vi "rmSharedMemory.vi"(8 "error in (no error)":errorcluster, 11 "SalProcess in":refnum<class "SalProcess.lvclass">) -> (0 "error out":errorcluster, 2 "outputMsg":string, 3 "SalProcess out":refnum<class "SalProcess.lvclass">)   [LabVIEW 2018, in "SalProcess.lvclass"]
doc: "Remove the shared memory of commandable SAL component (CSC)."
uses:
  SalProcess.lvclass
  SalProcess.lvclass/SalProcess.ctl
  LibReader/LibReader.lvclass/LibReader.ctl
  LibReader/LibReader.lvclass
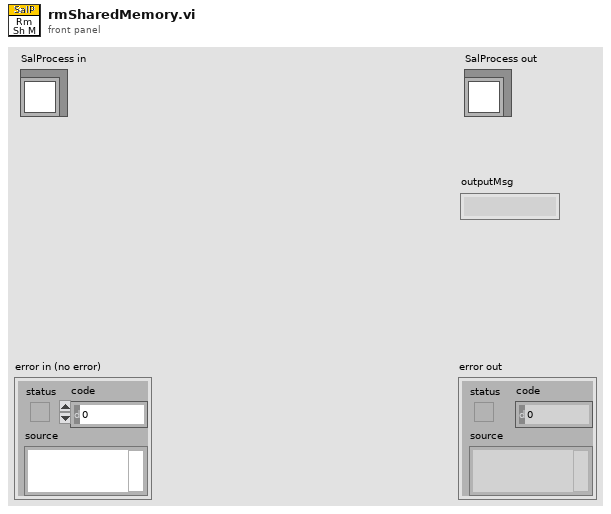
[diagram p1: front panel]
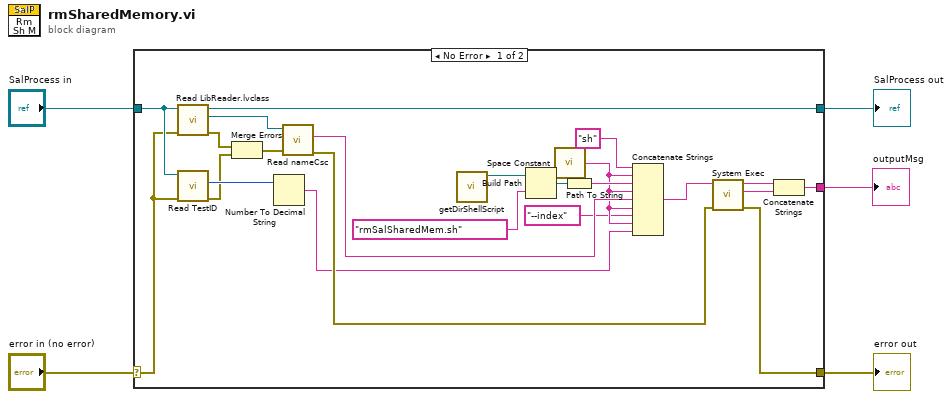
[diagram p0: block diagram]
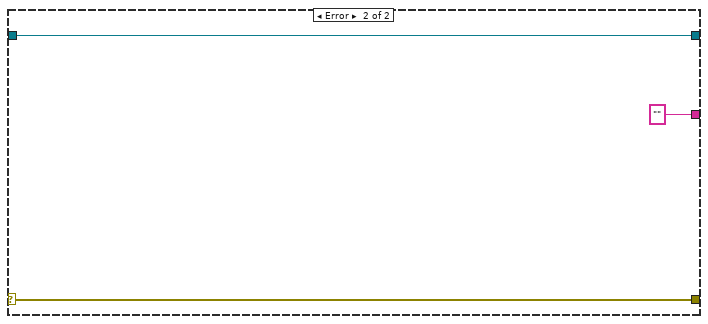
[diagram p2: hidden frame]
diagram:
  n1 = case shown="No Error" "error in (no error)" {
    selector: "error in (no error)" -> [w11 w31]
    tunnel: [w24 w31] -> w4
    tunnel: [w18 w30] -> w2
    tunnel: "SalProcess in" -> [w12 w30]
    tunnel: [w19 ""] -> w1
    frame No Error {
      n2 = call "Read LibReader.lvclass.vi"("error in (no error)"=w11, "SalProcess in"=w12) -> ("error out"=w7:errorcluster, "LibReader.lvclass"=w17:refnum<class "LibReader.lvclass">, "SalProcess out"=w18:refnum<class "SalProcess.lvclass">)  [unwired: 7 in]
      n3 = call "Read TestID.vi"("error in (no error)"=w11, "SalProcess in"=w12) -> ("error out"=w6:errorcluster, "TestID"=w10:i32)  [unwired: 7 in, 1 out]
      n4 = Merge Errors(w7, w6) -> (w8:errorcluster)
      n5 = Number To Decimal String(number=w10) -> (decimal integer string=w9:string)  [unwired: 1 in]
      n6 = call "Read nameCsc.vi"("error in (no error)"=w8, "LibReader in"=w17) -> ("error out"=w15:errorcluster, "nameCsc"=w16:string)  [unwired: 7 in, 1 out]
      n7 = call "getDirShellScript.vi"() -> ("dirShellScript"=w28:path)  [unwired: 11 in]
      n8 = Build Path(base path=w28, name or relative path="rmSalSharedMem.sh") -> (appended path=w26:path)
      n9 = call <vilib>:"Space Constant.vi"() -> ("String"=w14:string)
      n10 = Path To String(path=w26) -> (string=w25:string)
      n11 = Concatenate Strings("sh" ("string"), w14, w25, w14, w16, w14, "--index", w14, w9) -> (w22:string)
      n12 = call <vilib>:"System Exec.vi"("error in (no error)"=w15, "command line"=w22) -> ("error out"=w24:errorcluster, "standard error"=w20:string, "standard output"=w21:string)  [unwired: 6 in, 1 out]
      n13 = Concatenate Strings(w21, w20) -> (w19:string)
    }
    frame Error {
    }
  }
  "error out" <- w4
  "SalProcess out" <- w2
  "outputMsg" <- w1
